vi "test.vi"() -> ()   [LabVIEW 2024]
panel:
  out "XY Graph":cluster{dbl[], dbl[]}(graph)
  out "Y":dbl
  out "X":dbl
  in  "stop":bool
  out "read buffer":string
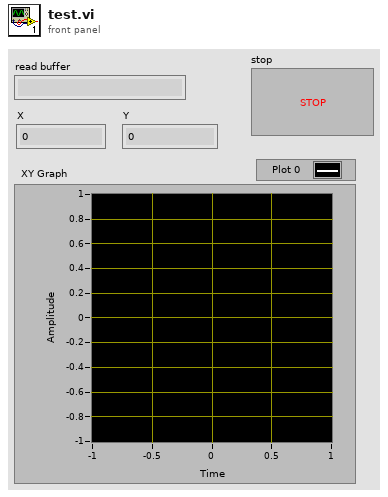
[diagram p1: front panel]
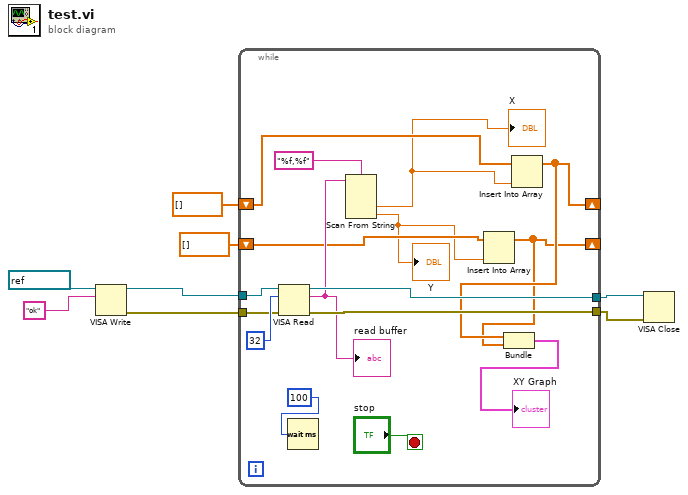
[diagram p0: block diagram]
diagram:
  n1 = VISA Write(VISA resource name=refnum<visa-resource-name> "COM8", write buffer="ok") -> (VISA resource name out=w1:refnum<visa-resource-name>, error out=w2:errorcluster)  [unwired: 1 in, 1 out]
  n2 = while {
    tunnel: [w20] -> w6
    tunnel: [w23] -> w5
    shift-right: [w15] -> _
    shift-left: dbl[] [] -> [w17]
    shift-right: [w14] -> _
    shift-left: dbl[] [] -> [w16]
    tunnel: w2 -> [w12]
    tunnel: w1 -> [w9]
    stop <- "stop" stop-if-true
    n3 = VISA Read(VISA resource name=w9, byte count=u32 32, error in (no error)=w12) -> (VISA resource name out=w20:refnum<visa-resource-name>, read buffer=w18:string, error out=w23:errorcluster)  [unwired: 1 out]
    "read buffer" <- w18
    n4 = Wait (ms)(milliseconds to wait=u32 100) -> ()  [unwired: 1 out]
    n5 = Scan From String(format string="%f,%f", input string=w18) -> (output 1=w11:dbl, output 2=w10:dbl)  [unwired: 4 in, 3 out]
    "X" <- w11
    "Y" <- w10
    n6 = Insert Into Array(array=w16, new element=w10) -> (w14:dbl[])  [unwired: 1 in]
    n7 = Insert Into Array(array=w17, new element=w11) -> (w15:dbl[])  [unwired: 1 in]
    n8 = Bundle(w15, w14) -> (→"XY Graph":cluster{dbl[], dbl[]})  [unwired: 1 in]
  }
  n9 = VISA Close(VISA resource name=w6, error in (no error)=w5) -> ()  [unwired: 1 out]
